vi "Do.vi"(8 "error in (no error)":errorcluster, 11 "Add Row to Database in":refnum<class "Add Row to Database.lvclass">) -> (0 "error out":errorcluster, 3 "Add Row to Database out":refnum<class "Add Row to Database.lvclass">)   [LabVIEW 2020, in "Panel Form Controller.lvlib" / "Add Row to Database.lvclass"]
uses:
  Add Row to Database.lvclass
  Add Row to Database.lvclass/Add Row to Database.ctl
  <vilib>/ActorFramework/Message Enqueuer/Message Enqueuer.lvclass/Message Enqueuer.ctl
  <vilib>/ActorFramework/Message Enqueuer/Enqueue.vi
  Panel Form Controller Messages/Add row to database Msg/Add row to database Msg.lvclass
  C:/Program Files (x86)/National Instruments/LabVIEW 2020/vi.lib/ActorFramework/Message/Message.lvclass
  <vilib>/ActorFramework/Message Priority Queue/Priority Enqueue.vi
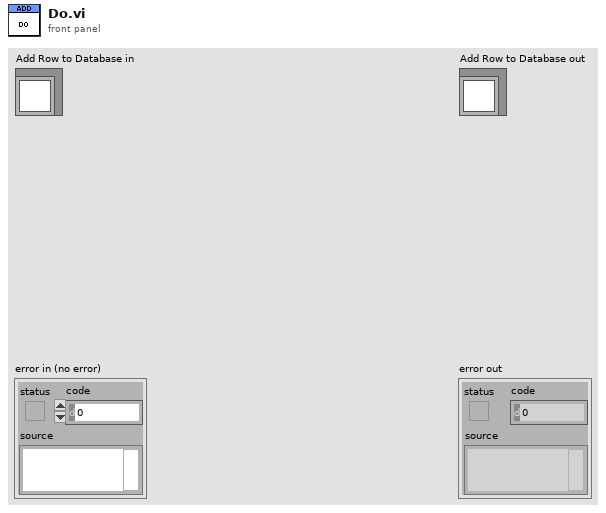
[diagram p1: front panel]
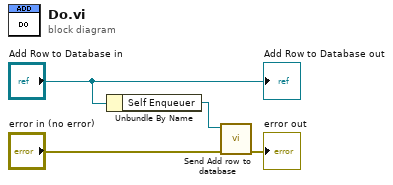
[diagram p0: block diagram]
diagram:
  n1 = Unbundle By Name("Add Row to Database in") -> ("Self Enqueuer"=w3:refnum<class "Message Enqueuer.lvclass">)
  n2 = call "Send Add row to database.vi"("error in (no error)"="error in (no error)", "Message Enqueuer"=w3) -> ("error out"=→"error out":errorcluster)  [unwired: 8 in, 1 out]
  "Add Row to Database out" <- "Add Row to Database in"
